vi "Read lines from file 2012NIVerified.vi"() -> ()   [LabVIEW 2018]
panel:
  in  "Stop Button":bool
  out "Text Lines":string[](array[string])
  in  "Read":bool
  in  "Lines to Read":i32
  in  "file path (use dialog)":path
  # "Overview: This code reads the number of lines specified in the chosen file.  Once the read has occurred,\nthe position within the file is reset to the beginning for this example.\nRequirements: LabVIEW 2012( (or compatible)\nInstructions:\n1. Run the vi.\n2. Specify the lines to read first\n3. Click on button\"Read\""
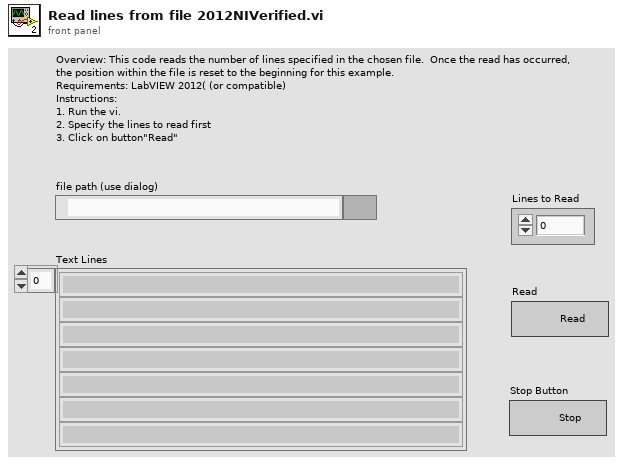
[diagram p1: front panel]
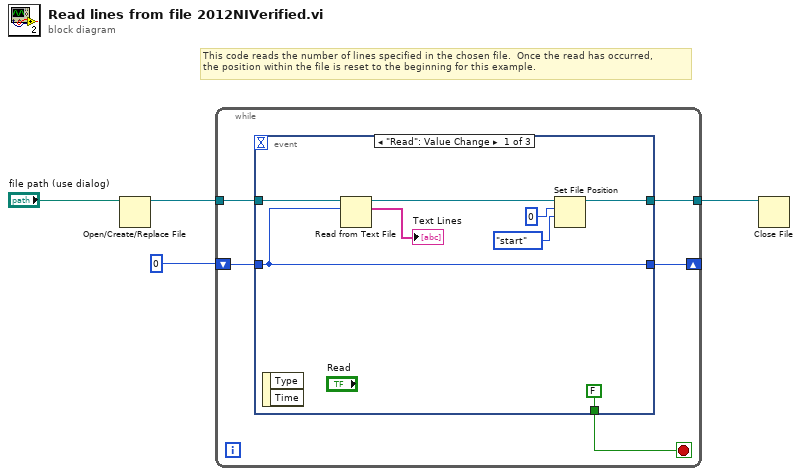
[diagram p0: block diagram]
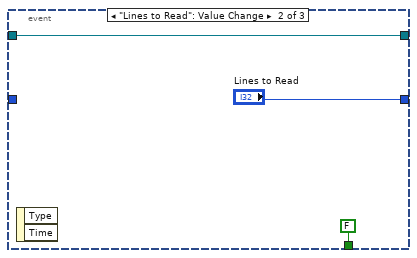
[diagram p2: hidden frame]
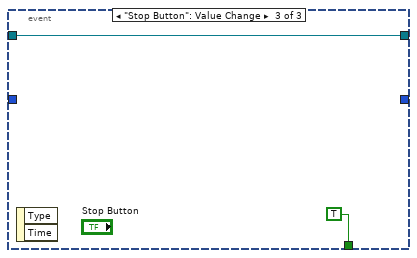
[diagram p3: hidden frame]
diagram:
  # "This code reads the number of lines specified in the chosen file.  Once the read has occurred,\nthe position within the file is reset to the beginning for this example."
  n1 = Open/Create/Replace File(file path (use dialog)="file path (use dialog)") -> (refnum out=w2:refnum<file>)  [unwired: 5 in, 2 out]
  n2 = while {
    shift-right: [w8] -> _
    shift-left: 0 -> [w9]
    tunnel: w2 -> [w6]
    tunnel: [w5] -> w1
    stop <- w7 stop-if-true
    n3 = event shown="[0] \"Read\": Value Change" {
      selector: _ -> [_ _ _]
      dyn-events: _ -> [_ _ _]
      timeout: _ -> [_ _ _]
      tunnel: w6 -> [w17 w19 w21]
      tunnel: w9 -> [w16 _ _]
      tunnel: [w16 "Lines to Read" _] -> w8
      tunnel: [w12 w19 w21] -> w5
      tunnel: [FALSE FALSE TRUE] -> w7
      event "Read": Value Change {
        n4 = event-data() -> ()  [unwired: 1 in, 2 out]
        n5 = Read from Text File(file (use dialog)=w17, count=w16) -> (refnum out=w13:refnum<file>, text=→"Text Lines":string[])  [unwired: 2 in, 2 out]
        n6 = Set File Position(offset (in bytes) (0)=i64 0, refnum=w13, from (0:start)=enum16{"start", "end", "current"}."start") -> (refnum out=w12:refnum<file>)  [unwired: 1 in, 1 out]
      }
      event "Lines to Read": Value Change {
        n7 = event-data() -> ()  [unwired: 1 in, 2 out]
      }
      event "Stop Button": Value Change {
        n8 = event-data() -> ()  [unwired: 1 in, 2 out]
      }
    }
  }
  n9 = Close File(refnum=w1) -> ()  [unwired: 1 in, 2 out]
